vi "KP_lab1.vi"() -> ()   [LabVIEW 2025]
panel:
  out "XY Graph 2":T1(graph)
  out "HEART RATE ZONES":string[][](array[string])
  out "BPM":cluster{"Time":timestamp[], "Bpm":i32[]}(graph)
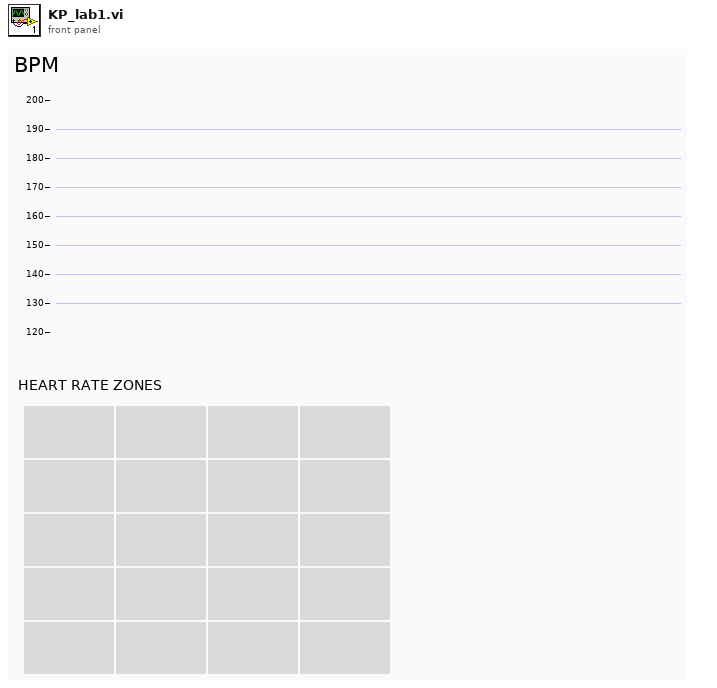
[diagram p1: front panel]
types:
  T1 = cluster{" Total time in Zone (%) ":dbl[], "Heart Rate Zone":i32[]}
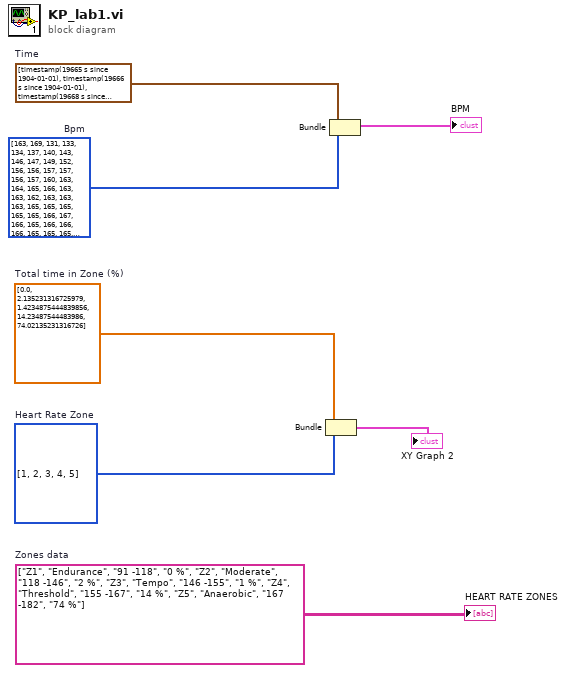
[diagram p0: block diagram]
diagram:
  w3 = timestamp[] [timestamp(19665 s since 1904-01-01), timestamp(19666 s since 1904-01-01), timestamp(19668 s since 1904-01-01), timestamp(19670 s since 1904-01-01), timestamp(19673 s since 1904-01-01), timestamp(19675 s since 1904-01-01), timestamp(19677 s since 1904-01-01), timestamp(19678 s since 1904-01-01), timestamp(19680 s since 1904-01-01), timestamp(19683 s since 1904-01-01), timestamp(19688 s since 1904-01-01), timestamp(19689 s since 1904-01-01), timestamp(19694 s since 1904-01-01), timestamp(19697 s since 1904-01-01), timestamp(19700 s since 1904-01-01), timestamp(19704 s since 1904-01-01), timestamp(19708 s since 1904-01-01), timestamp(19713 s since 1904-01-01), timestamp(19718 s since 1904-01-01), timestamp(19720 s since 1904-01-01), timestamp(19724 s since 1904-01-01), timestamp(19730 s since 1904-01-01), timestamp(19731 s since 1904-01-01), timestamp(19737 s since 1904-01-01), timestamp(19740 s since 1904-01-01), timestamp(19746 s since 1904-01-01), timestamp(19747 s since 1904-01-01), timestamp(19753 s since 1904-01-01), timestamp(19754 s since 1904-01-01), timestamp(19760 s since 1904-01-01), timestamp(19763 s since 1904-01-01), timestamp(19768 s since 1904-01-01), timestamp(19774 s since 1904-01-01), timestamp(19780 s since 1904-01-01), timestamp(19783 s since 1904-01-01), timestamp(19789 s since 1904-01-01), timestamp(19793 s since 1904-01-01), timestamp(19797 s since 1904-01-01), timestamp(19801 s since 1904-01-01), timestamp(19807 s since 1904-01-01), timestamp(19810 s since 1904-01-01), timestamp(19816 s since 1904-01-01), timestamp(19817 s since 1904-01-01), timestamp(19819 s since 1904-01-01), timestamp(19823 s since 1904-01-01), timestamp(19829 s since 1904-01-01), timestamp(19830 s since 1904-01-01), timestamp(19836 s since 1904-01-01), timestamp(19838 s since 1904-01-01), timestamp(19842 s since 1904-01-01), timestamp(19848 s since 1904-01-01), timestamp(19854 s since 1904-01-01), timestamp(19855 s since 1904-01-01), timestamp(19861 s since 1904-01-01), timestamp(19866 s since 1904-01-01), timestamp(19871 s since 1904-01-01), timestamp(19877 s since 1904-01-01), timestamp(19878 s since 1904-01-01), timestamp(19884 s since 1904-01-01), timestamp(19887 s since 1904-01-01), timestamp(19890 s since 1904-01-01), timestamp(19896 s since 1904-01-01), timestamp(19902 s since 1904-01-01), timestamp(19903 s since 1904-01-01), timestamp(19906 s since 1904-01-01), timestamp(19910 s since 1904-01-01), timestamp(19916 s since 1904-01-01), timestamp(19918 s since 1904-01-01), timestamp(19923 s since 1904-01-01), timestamp(19925 s since 1904-01-01), timestamp(19926 s since 1904-01-01), timestamp(19932 s since 1904-01-01), timestamp(19933 s since 1904-01-01), timestamp(19939 s since 1904-01-01), timestamp(19940 s since 1904-01-01), timestamp(19946 s since 1904-01-01), timestamp(19949 s since 1904-01-01), timestamp(19955 s since 1904-01-01), timestamp(19957 s since 1904-01-01), timestamp(19963 s since 1904-01-01), timestamp(19969 s since 1904-01-01), timestamp(19975 s since 1904-01-01), timestamp(19978 s since 1904-01-01), timestamp(19984 s since 1904-01-01), timestamp(19986 s since 1904-01-01), timestamp(19992 s since 1904-01-01), timestamp(19994 s since 1904-01-01), timestamp(20000 s since 1904-01-01), timestamp(20005 s since 1904-01-01), timestamp(20009 s since 1904-01-01), timestamp(20014 s since 1904-01-01), timestamp(20016 s since 1904-01-01), timestamp(20022 s since 1904-01-01), timestamp(20024 s since 1904-01-01), timestamp(20025 s since 1904-01-01), timestamp(20031 s since 1904-01-01), timestamp(20033 s since 1904-01-01), timestamp(20038 s since 1904-01-01), timestamp(20042 s since 1904-01-01), timestamp(20047 s since 1904-01-01), timestamp(20049 s since 1904-01-01), timestamp(20055 s since 1904-01-01), timestamp(20057 s since 1904-01-01), timestamp(20062 s since 1904-01-01), timestamp(20063 s since 1904-01-01), timestamp(20068 s since 1904-01-01), timestamp(20070 s since 1904-01-01), timestamp(20075 s since 1904-01-01), timestamp(20077 s since 1904-01-01), timestamp(20083 s since 1904-01-01), timestamp(20085 s since 1904-01-01), timestamp(20090 s since 1904-01-01), timestamp(20092 s since 1904-01-01), timestamp(20098 s since 1904-01-01), timestamp(20099 s since 1904-01-01), timestamp(20104 s since 1904-01-01), timestamp(20109 s since 1904-01-01), timestamp(20114 s since 1904-01-01), timestamp(20115 s since 1904-01-01), timestamp(20121 s since 1904-01-01), timestamp(20124 s since 1904-01-01), timestamp(20130 s since 1904-01-01), timestamp(20132 s since 1904-01-01), timestamp(20137 s since 1904-01-01), timestamp(20142 s since 1904-01-01), timestamp(20145 s since 1904-01-01), timestamp(20151 s since 1904-01-01), timestamp(20152 s since 1904-01-01), timestamp(20153 s since 1904-01-01), timestamp(20159 s since 1904-01-01), timestamp(20160 s since 1904-01-01), timestamp(20166 s since 1904-01-01), timestamp(20167 s since 1904-01-01), timestamp(20173 s since 1904-01-01), timestamp(20176 s since 1904-01-01), timestamp(20181 s since 1904-01-01), timestamp(20184 s since 1904-01-01), timestamp(20190 s since 1904-01-01), timestamp(20192 s since 1904-01-01), timestamp(20198 s since 1904-01-01), timestamp(20203 s since 1904-01-01), timestamp(20205 s since 1904-01-01), timestamp(20210 s since 1904-01-01), timestamp(20216 s since 1904-01-01), timestamp(20218 s since 1904-01-01), timestamp(20224 s since 1904-01-01), timestamp(20227 s since 1904-01-01), timestamp(20233 s since 1904-01-01), timestamp(20235 s since 1904-01-01), timestamp(20241 s since 1904-01-01), timestamp(20242 s since 1904-01-01), timestamp(20248 s since 1904-01-01), timestamp(20253 s since 1904-01-01), timestamp(20259 s since 1904-01-01), timestamp(20261 s since 1904-01-01), timestamp(20267 s since 1904-01-01), timestamp(20270 s since 1904-01-01), timestamp(20276 s since 1904-01-01), timestamp(20278 s since 1904-01-01), timestamp(20284 s since 1904-01-01), timestamp(20288 s since 1904-01-01), timestamp(20294 s since 1904-01-01), timestamp(20296 s since 1904-01-01), timestamp(20302 s since 1904-01-01), timestamp(20304 s since 1904-01-01), timestamp(20310 s since 1904-01-01), timestamp(20311 s since 1904-01-01), timestamp(20317 s since 1904-01-01), timestamp(20319 s since 1904-01-01), timestamp(20325 s since 1904-01-01), timestamp(20326 s since 1904-01-01), timestamp(20332 s since 1904-01-01), timestamp(20333 s since 1904-01-01), timestamp(20339 s since 1904-01-01), timestamp(20343 s since 1904-01-01), timestamp(20349 s since 1904-01-01), timestamp(20350 s since 1904-01-01), timestamp(20356 s since 1904-01-01), timestamp(20357 s since 1904-01-01), timestamp(20360 s since 1904-01-01), timestamp(20366 s since 1904-01-01), timestamp(20367 s since 1904-01-01), timestamp(20373 s since 1904-01-01), timestamp(20374 s since 1904-01-01), timestamp(20379 s since 1904-01-01), timestamp(20380 s since 1904-01-01), timestamp(20385 s since 1904-01-01), timestamp(20386 s since 1904-01-01), timestamp(20392 s since 1904-01-01), timestamp(20397 s since 1904-01-01), timestamp(20399 s since 1904-01-01), timestamp(20404 s since 1904-01-01), timestamp(20408 s since 1904-01-01), timestamp(20414 s since 1904-01-01), timestamp(20417 s since 1904-01-01), timestamp(20423 s since 1904-01-01), timestamp(20427 s since 1904-01-01), timestamp(20433 s since 1904-01-01), timestamp(20438 s since 1904-01-01), timestamp(20441 s since 1904-01-01), timestamp(20442 s since 1904-01-01), timestamp(20442 s since 1904-01-01), timestamp(20447 s since 1904-01-01), timestamp(20449 s since 1904-01-01), timestamp(20454 s since 1904-01-01), timestamp(20458 s since 1904-01-01), timestamp(20464 s since 1904-01-01), timestamp(20466 s since 1904-01-01), timestamp(20471 s since 1904-01-01), timestamp(20476 s since 1904-01-01), timestamp(20482 s since 1904-01-01), timestamp(20488 s since 1904-01-01), timestamp(20490 s since 1904-01-01), timestamp(20496 s since 1904-01-01), timestamp(20498 s since 1904-01-01), timestamp(20504 s since 1904-01-01), timestamp(20509 s since 1904-01-01), timestamp(20511 s since 1904-01-01), timestamp(20513 s since 1904-01-01), timestamp(20517 s since 1904-01-01), timestamp(20522 s since 1904-01-01), timestamp(20525 s since 1904-01-01), timestamp(20530 s since 1904-01-01), timestamp(20531 s since 1904-01-01), timestamp(20537 s since 1904-01-01), timestamp(20539 s since 1904-01-01), timestamp(20545 s since 1904-01-01), timestamp(20546 s since 1904-01-01), timestamp(20552 s since 1904-01-01), timestamp(20553 s since 1904-01-01), timestamp(20558 s since 1904-01-01), timestamp(20559 s since 1904-01-01), timestamp(20562 s since 1904-01-01), timestamp(20565 s since 1904-01-01), timestamp(20570 s since 1904-01-01), timestamp(20575 s since 1904-01-01), timestamp(20580 s since 1904-01-01), timestamp(20581 s since 1904-01-01), timestamp(20586 s since 1904-01-01), timestamp(20591 s since 1904-01-01), timestamp(20597 s since 1904-01-01), timestamp(20600 s since 1904-01-01), timestamp(20605 s since 1904-01-01), timestamp(20606 s since 1904-01-01), timestamp(20610 s since 1904-01-01), timestamp(20613 s since 1904-01-01), timestamp(20614 s since 1904-01-01), timestamp(20616 s since 1904-01-01), timestamp(20621 s since 1904-01-01), timestamp(20622 s since 1904-01-01), timestamp(20627 s since 1904-01-01), timestamp(20628 s since 1904-01-01), timestamp(20634 s since 1904-01-01), timestamp(20638 s since 1904-01-01), timestamp(20643 s since 1904-01-01), timestamp(20644 s since 1904-01-01), timestamp(20648 s since 1904-01-01), timestamp(20652 s since 1904-01-01), timestamp(20653 s since 1904-01-01), timestamp(20655 s since 1904-01-01), timestamp(20660 s since 1904-01-01), timestamp(20666 s since 1904-01-01), timestamp(20667 s since 1904-01-01), timestamp(20673 s since 1904-01-01), timestamp(20678 s since 1904-01-01), timestamp(20684 s since 1904-01-01), timestamp(20690 s since 1904-01-01), timestamp(20691 s since 1904-01-01), timestamp(20694 s since 1904-01-01), timestamp(20697 s since 1904-01-01), timestamp(20698 s since 1904-01-01)]  # Time
  w2 = i32[] [163, 169, 131, 133, 134, 137, 140, 143, 146, 147, 149, 152, 156, 156, 157, 157, 156, 157, 160, 163, 164, 165, 166, 163, 163, 162, 163, 163, 163, 165, 165, 165, 165, 165, 166, 167, 166, 165, 166, 166, 166, 165, 165, 165, 166, 166, 166, 164, 164, 165, 165, 166, 167, 167, 167, 167, 168, 168, 168, 168, 167, 167, 167, 168, 167, 167, 167, 168, 169, 168, 169, 169, 168, 173, 176, 170, 169, 170, 170, 170, 170, 171, 172, 172, 172, 171, 171, 171, 171, 172, 173, 173, 173, 173, 173, 173, 172, 173, 173, 172, 172, 173, 172, 173, 173, 173, 173, 172, 172, 172, 173, 172, 173, 172, 173, 174, 173, 174, 174, 173, 173, 173, 174, 173, 172, 173, 173, 173, 174, 173, 174, 174, 173, 174, 174, 176, 175, 175, 175, 174, 177, 180, 175, 175, 175, 175, 175, 176, 174, 174, 174, 175, 175, 175, 175, 175, 174, 174, 176, 177, 176, 176, 176, 176, 177, 176, 177, 177, 176, 176, 176, 177, 177, 177, 177, 178, 178, 177, 176, 177, 176, 177, 177, 177, 177, 177, 177, 177, 178, 177, 178, 178, 178, 177, 176, 178, 178, 179, 178, 178, 178, 179, 180, 179, 180, 180, 179, 180, 184, 179, 180, 179, 179, 179, 179, 179, 179, 180, 179, 179, 180, 179, 178, 179, 179, 179, 179, 180, 180, 180, 180, 180, 180, 179, 179, 179, 179, 179, 179, 179, 180, 178, 180, 180, 180, 180, 180, 180, 181, 180, 180, 179, 181, 181, 181, 181, 182, 182, 182, 181, 182, 182, 182, 182, 182, 182, 182, 181, 181, 182, 183, 183, 182, 183, 184, 183, 183, 183, 184, 183, 184]  # Bpm
  w5 = dbl[] [0.0, 2.135231316725979, 1.4234875444839856, 14.23487544483986, 74.02135231316726]  # Total time in Zone (%)
  w7 = string[][] [["Z1", "Endurance", "91 -118", "0 %"], ["Z2", "Moderate", "118 -146", "2 %"], ["Z3", "Tempo", "146 -155", "1 %"], ["Z4", "Threshold", "155 -167", "14 %"], ["Z5", "Anaerobic", "167 -182", "74 %"]]  # Zones data
  w6 = i32[] [1, 2, 3, 4, 5]  # Heart Rate Zone
  n1 = Bundle("Total time in Zone (%)"=w5, "Heart Rate Zone"=w6) -> (→"XY Graph 2":T1)  [unwired: 1 in]
  n2 = Bundle("Time"=w3, "Bpm"=w2) -> (→"BPM":cluster{"Time":timestamp[], "Bpm":i32[]})  [unwired: 1 in]
  "HEART RATE ZONES" <- w7
